vi "Seq Dialog Check Digital Input MCAS.vi"(8 "Segment Data":T4) -> (0 "Step Hisitory":string[](array[string]), 2 "Segment Data 2":T4)   [LabVIEW 2018]
uses:
  type defs/Sequence Info.ctl
  type defs/MCAS Digital Input Control_single nest.ctl
  type defs/misc digital input.ctl
  type defs/MCAS Digital Input Cluster Control 1.ctl
  type defs/Digital Input Pointer.ctl
panel:
  in  "Nest Index":i32=1 min=1 step=1
  in  "Misc Input":T1
  in  "Station Digital Input":T2
  in  "input type":T3(radio)
  in  "Boolean":bool
  out "Name":string="Pre Run Station - Glass - Vent Open"
  in  "Description":string
  in  "Save":bool
  in  "Cancel":bool
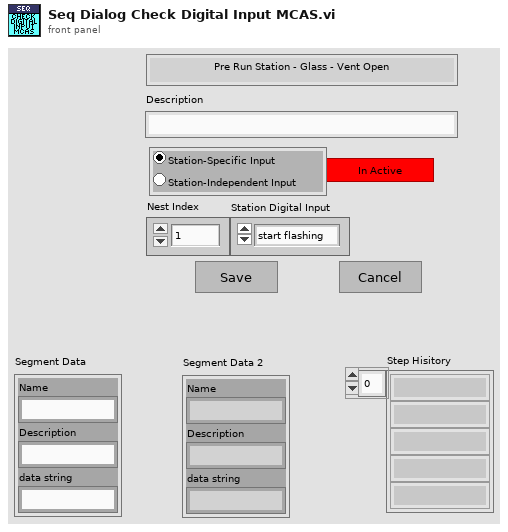
[diagram p1: front panel]
types:
  T1 = typedef "misc digital input.ctl" = enum16{"part select bit 0", "part select bit 1", "part select bit 2", "part select bit 3"}
  T2 = typedef "MCAS Digital Input Control_single nest.ctl" = enum16{"start flashing", "reject", "part present 1", "part present 2", "clamp opened", "clamp closed", "tool select bit 0", "tool select bit 1"}
  T3 = enum32{"Station-Specific Input", "Station-Independent Input"}
  T4 = typedef "Sequence Info.ctl" = cluster{"Name":string, "Description":string, "data string":string}
  T5 = typedef "MCAS Digital Input Cluster Control 1.ctl" = cluster{"Status":bool, "Digital Input":T6}
  T6 = typedef "Digital Input Pointer.ctl" = cluster{"Station Digital Input":T2, "Station Index":i32, "Misc Input":T1}
  T7 = cluster{"Segment Data":T4, "Old Data":string, "New Data":string, "MCFS Digital Input Cluster":T5}
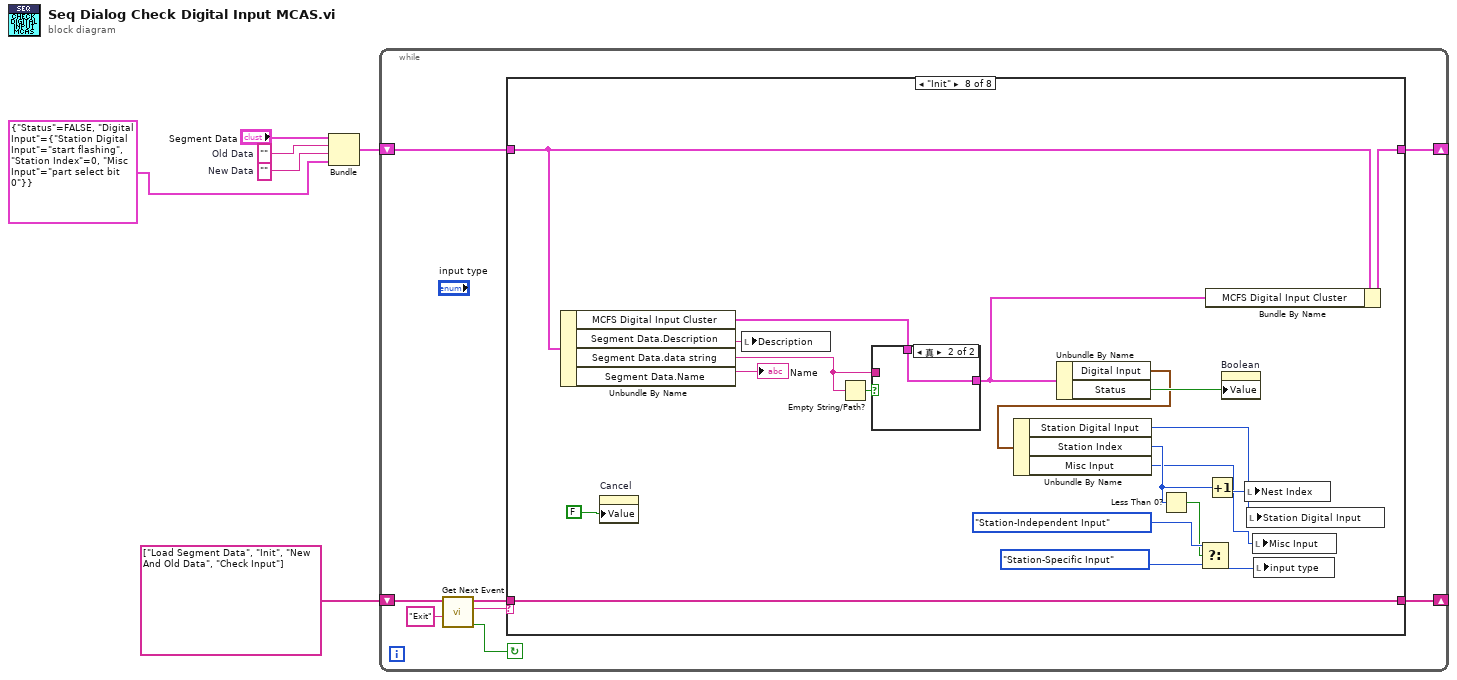
[diagram p0: block diagram]
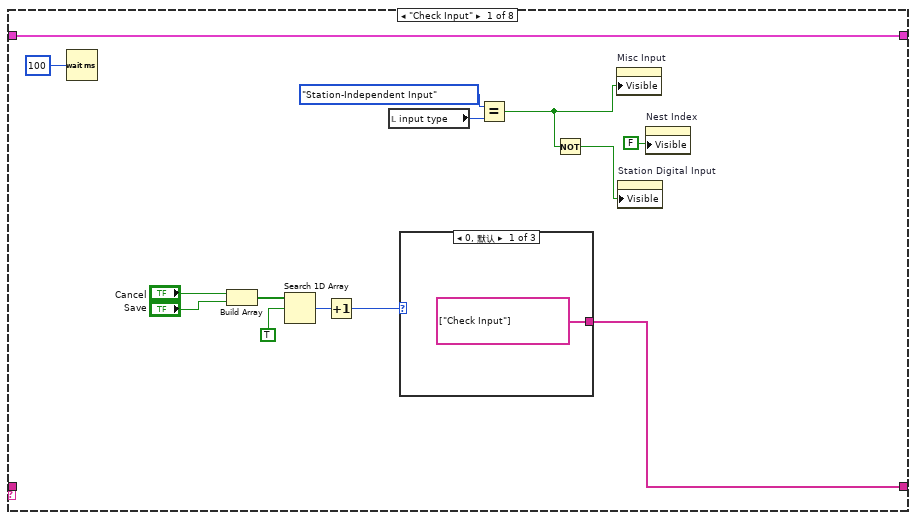
[diagram p2: hidden frame]
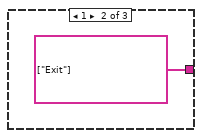
[diagram p3: hidden frame]
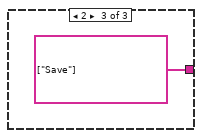
[diagram p4: hidden frame]
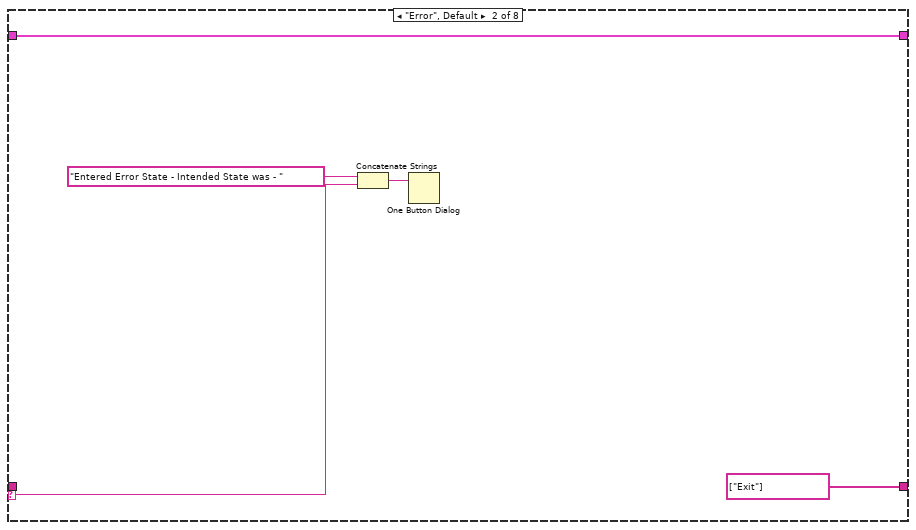
[diagram p5: hidden frame]
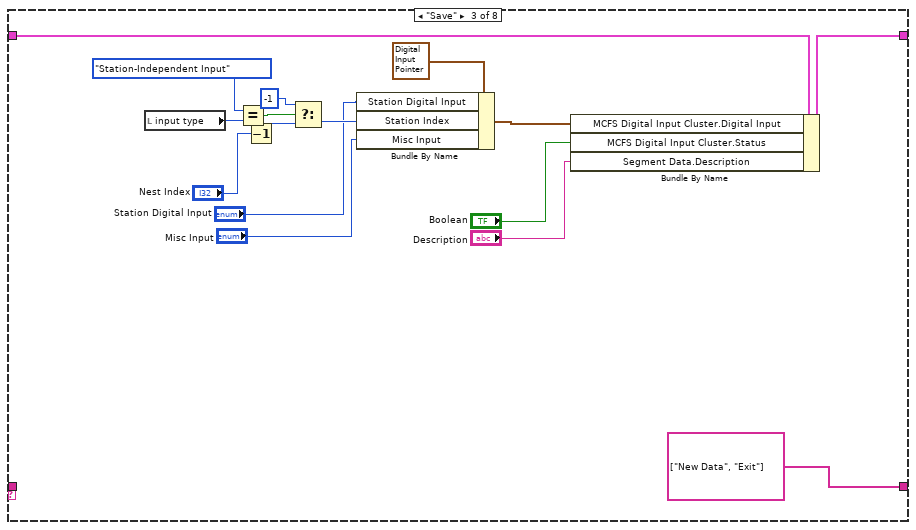
[diagram p6: hidden frame]
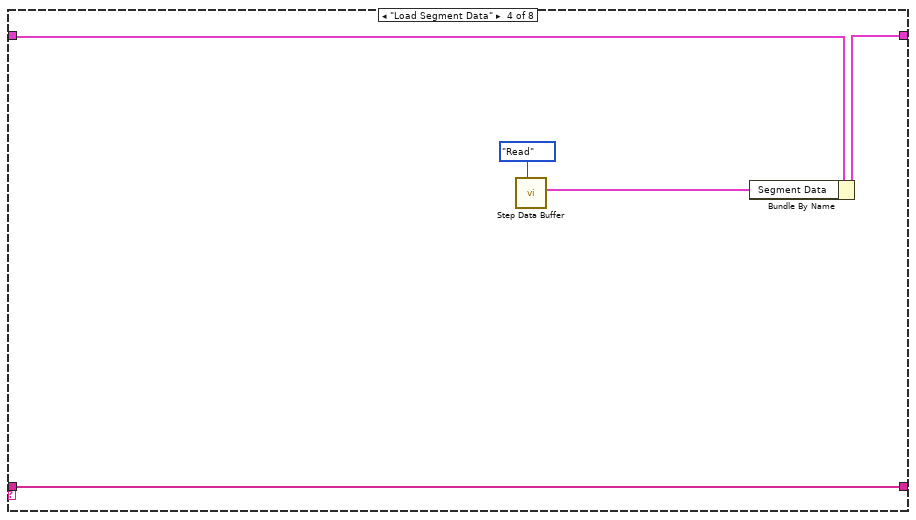
[diagram p7: hidden frame]
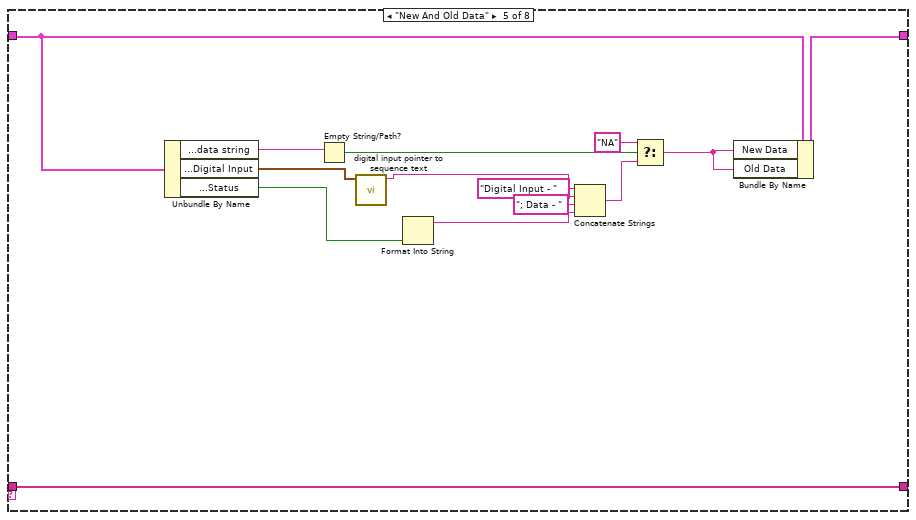
[diagram p8: hidden frame]
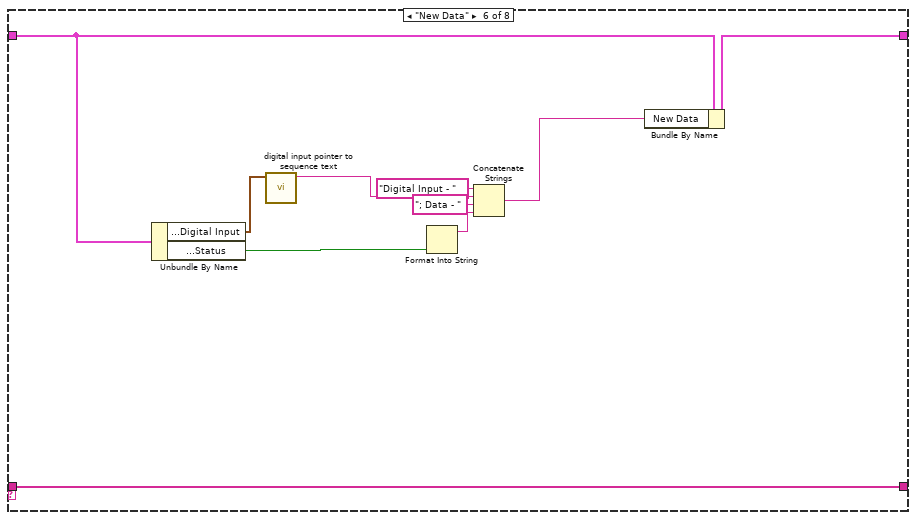
[diagram p9: hidden frame]
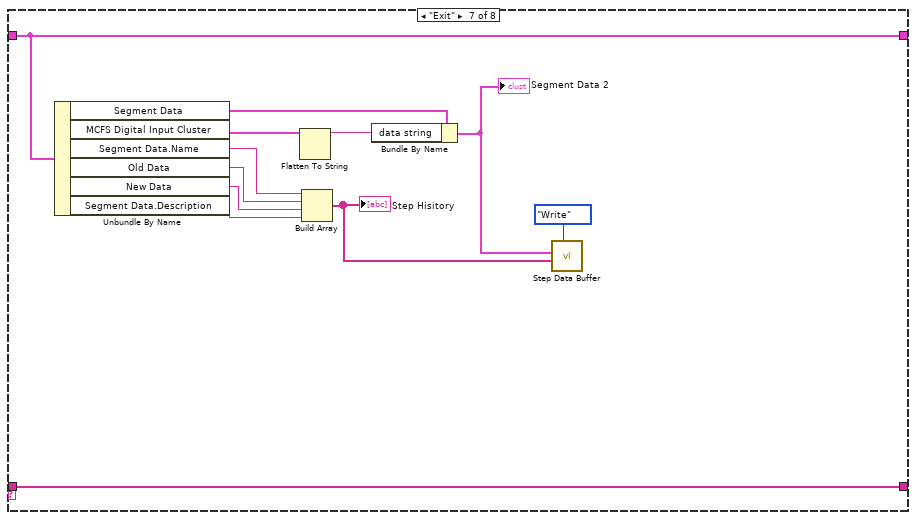
[diagram p10: hidden frame]
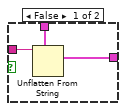
[diagram p11: hidden frame]
diagram:
  w3 = ""  # New Data
  w4 = ""  # Old Data
  n1 = Bundle("Segment Data"="Segment Data", "Old Data"=w4, "New Data"=w3, "MCFS Digital Input Cluster"=T5 {"Status"=FALSE, "Digital Input"={"Station Digital Input"=enum."start flashing", "Station Index"=0, "Misc Input"=enum."part select bit 0"}}) -> (w6:T7)  [unwired: 1 in]
  n2 = while {
    shift-right: [w12] -> _
    shift-left: string[] ["Load Segment Data", "Init", "New And Old Data", "Check Input"] ("Event queue out") -> [w11]
    shift-right: [w7] -> _
    shift-left: w6 -> [w8]
    stop <- w10 continue-if-true
    n3 = call "Get Next Event.vi"("Exit Event"="Exit", "event queue in"=w11) -> ("Condition (Exit:F)"=w10:bool, "next event"=w14:string, "event queue out"=w13:string[])  [unwired: 3 in]
    n4 = case shown="\"Init\"" w14 {
      selector: w14 -> [_ w34 _ _ _ _ _ _]
      tunnel: w13 -> [_ _ _ w53 w65 w81 w93 w113]
      tunnel: [w22 string[] ["Exit"] ("event queue out") string[] ["New Data", "Exit"] ("Event queue out") w53 w65 w81 w93 w113] -> w12
      tunnel: w8 -> [w27 w32 w51 w55 w67 w80 w92 w108]
      tunnel: [w27 w32 w52 w54 w66 w79 w92 w105] -> w7
      frame "Check Input" {
        n5 = Wait (ms)(milliseconds to wait=u32 100) -> ()  [unwired: 1 out]
        n6 = Build Array("Cancel", "Save") -> (w24:bool[])
        n7 = Search 1D Array(1D array=w24, element=TRUE) -> (index of element=w25:i32)  [unwired: 1 in]
        n8 = Increment(x=w25) -> (x+1=w26:i32)
        n9 = local read "input type"() -> (w19:T3)
        n10 = case shown="0, 默认" w26 {
          tunnel: [string[] ["Check Input"] ("Events to Insert") string[] ["Exit"] ("Events to Insert") string[] ["Save"] ("Events to Insert")] -> w22
          frame 0, Default {
          }
          frame 1 {
          }
          frame 2 {
          }
        }
        n11 = Equal?(x=T3."Station-Independent Input", y=w19) -> (x = y?=w17:bool)
        n12 = Not(x=w17) -> (.not. x?=w16:bool)
        n13 = property on="Misc Input" class="Enum (严格)"("Visible"=w17) -> ()  [unwired: 2 in, 2 out]
        n14 = property on="Station Digital Input" class="Enum (严格)"("Visible"=w16) -> ()  [unwired: 2 in, 2 out]
        n15 = property on="Nest Index" class="DigNum (严格)"("Visible"=FALSE) -> ()  [unwired: 2 in, 2 out]
      }
      frame "Error", Default {
        n16 = Concatenate Strings("Entered Error State - Intended State was - " ("string"), w34) -> (w36:string)
        n17 = One Button Dialog(message=w36) -> ()  [unwired: 1 in, 1 out]
      }
      frame "Save" {
        n18 = local read "input type"() -> (w40:T3)
        n19 = Equal?(x=T3."Station-Independent Input", y=w40) -> (x = y?=w43:bool)
        n20 = Decrement(x="Nest Index") -> (x-1=w45:i32)
        n21 = Select(t=-1, s=w43, f=w45) -> (s? t:f=w42:i32)
        n22 = Bundle By Name(cluster=T6 {"Station Digital Input"=enum."start flashing", "Station Index"=0, "Misc Input"=enum."part select bit 0"} ("Digital Input"), "Station Digital Input"="Station Digital Input", "Station Index"=w42, "Misc Input"="Misc Input") -> (w46:T6)
        n23 = Bundle By Name(cluster=w51, "MCFS Digital Input Cluster.Digital Input"=w46, "MCFS Digital Input Cluster.Status"="Boolean", "Segment Data.Description"="Description") -> (w52:T7)
      }
      frame "Load Segment Data" {
        n24 = call "Step Data Buffer.vi"("Mode"=enum16{"Init", "Read", "Write"}."Read") -> ("Segment Data Out"=w57:T4)  [unwired: 6 in, 4 out]
        n25 = Bundle By Name(cluster=w55, "Segment Data"=w57) -> (w54:T7)
      }
      frame "New And Old Data" {
        n26 = Unbundle By Name(w67) -> ("Segment Data.data string"=w71:string, "MCFS Digital Input Cluster.Digital Input"=w59:T6, "MCFS Digital Input Cluster.Status"=w61:bool)
        n27 = Empty String/Path?(string/path=w71) -> (empty?=w68:bool)
        n28 = call "digital input pointer to sequence text.vi"("Digital Input"=w59) -> ("String"=w58:string)  [unwired: 10 in]
        n29 = Format Into String(w61) -> (resulting string=w60:string)  [unwired: 3 in, 1 out]
        n30 = Concatenate Strings("Digital Input - " ("string"), w58, "; Data - " ("string"), w60) -> (w62:string)
        n31 = Select(t="NA", s=w68, f=w62) -> (s? t:f=w70:string)
        n32 = Bundle By Name(cluster=w67, "New Data"=w70, "Old Data"=w70) -> (w66:T7)
      }
      frame "New Data" {
        n33 = Unbundle By Name(w80) -> ("MCFS Digital Input Cluster.Digital Input"=w73:T6, "MCFS Digital Input Cluster.Status"=w75:bool)
        n34 = call "digital input pointer to sequence text.vi"("Digital Input"=w73) -> ("String"=w72:string)  [unwired: 10 in]
        n35 = Format Into String(w75) -> (resulting string=w74:string)  [unwired: 3 in, 1 out]
        n36 = Concatenate Strings("Digital Input - " ("string"), w72, "; Data - " ("string"), w74) -> (w76:string)
        n37 = Bundle By Name(cluster=w80, "New Data"=w76) -> (w79:T7)
      }
      frame "Exit" {
        n38 = Unbundle By Name(w92) -> ("Segment Data"=w85:T4, "MCFS Digital Input Cluster"=w83:T5, "Segment Data.Name"=w91:string, "Old Data"=w90:string, "New Data"=w89:string, "Segment Data.Description"=w86:string)
        n39 = Flatten To String(anything=w83) -> (data string=w82:string)  [unwired: 3 in, 2 out]
        n40 = Build Array(w91, w90, w89, w86) -> (w87:string[])
        "Step Hisitory" <- w87
        n41 = Bundle By Name(cluster=w85, "data string"=w82) -> (w84:T4)
        "Segment Data 2" <- w84
        n42 = call "Step Data Buffer.vi"("Mode"=enum16{"Init", "Read", "Write"}."Write", "Step Hisitory In"=w87, "Segment Data In"=w84) -> ()  [unwired: 4 in, 5 out]
      }
      frame "Init" {
        n43 = Unbundle By Name(w108) -> ("MCFS Digital Input Cluster"=w109:T5, "Segment Data.Description"=w112:string, "Segment Data.data string"=w106:string, "Segment Data.Name"=→"Name":string)
        n44 = property on="Cancel" class="Bool (严格)"("Value"=FALSE ("Cancel")) -> ()  [unwired: 2 in, 2 out]
        n45 = local write "Description"(w112) -> ()
        n46 = Empty String/Path?(string/path=w106) -> (empty?=w107:bool)
        n47 = case shown="真" w107 {
          tunnel: w106 -> [w116 _]
          tunnel: w109 -> [w115 w117]
          tunnel: [w114 w117] -> w103
          frame False {
            n48 = Unflatten From String(type=w115, binary string=w116) -> (value=w114:T5)  [unwired: 3 in, 2 out]
          }
          frame True {
          }
        }
        n49 = Unbundle By Name(w103) -> ("Digital Input"=w98:T6, "Status"=w104:bool)
        n50 = Unbundle By Name(w98) -> ("Station Digital Input"=w95:T2, "Station Index"=w96:i32, "Misc Input"=w94:T1)
        n51 = Less Than 0?(x=w96) -> (x < 0?=w99:bool)
        n52 = Select(t=T3."Station-Independent Input" ("input type"), s=w99, f=T3."Station-Specific Input" ("input type")) -> (s? t:f=w102:T3)
        n53 = Bundle By Name(cluster=w108, "MCFS Digital Input Cluster"=w103) -> (w105:T7)
        n54 = Increment(x=w96) -> (x+1=w97:i32)
        n55 = property on="Boolean" class="Bool (严格)"("Value"=w104) -> ()  [unwired: 2 in, 2 out]
        n56 = local write "Nest Index"(w97) -> ()
        n57 = local write "Station Digital Input"(w95) -> ()
        n58 = local write "Misc Input"(w94) -> ()
        n59 = local write "input type"(w102) -> ()
      }
    }
  }
